vi "MDAQ_WRITE.vi"(8 "error in":errorcluster, 9 "ARG":string, 10 "CMD":string, 11 "VISA resource name":refnum<visa-resource-name>) -> (0 "error out":errorcluster, 3 "VISA resource name out":refnum<visa-resource-name>)   [LabVIEW 2021]
uses:
  e2ee38f0-3462-4155-9d7d-371542cbdf2c.vi
  e0b7c9b4-ca0d-4614-8169-0355f0fe5c3c.vi
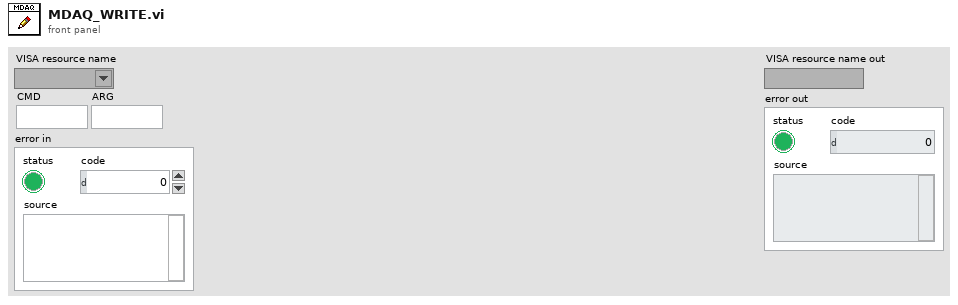
[diagram p1: front panel]
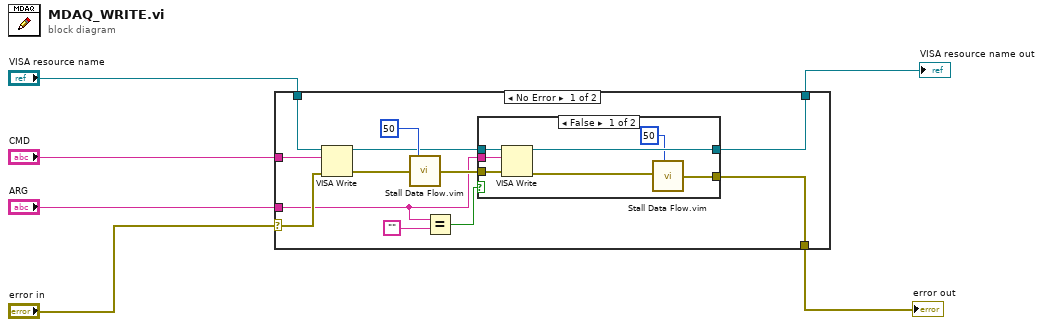
[diagram p0: block diagram]
diagram:
  n1 = case shown="No Error" "error in" {
    selector: "error in" -> [w12 w28]
    tunnel: "VISA resource name" -> [w18 w29]
    tunnel: "CMD" -> [w17 _]
    tunnel: "ARG" -> [w11 _]
    tunnel: [w8 w29] -> w3
    tunnel: [w7 w28] -> w2
    frame No Error {
      n2 = VISA Write(VISA resource name=w18, write buffer=w17, error in (no error)=w12) -> (VISA resource name out=w14:refnum<visa-resource-name>, error out=w16:errorcluster)  [unwired: 1 out]
      n3 = call "Stall Data Flow.vim"("value in"=w16, "milliseconds to wait"=u32 50) -> ("value out"=w13:errorcluster)  [unwired: 1 out]
      n4 = Equal?(x=w11, y="") -> (x = y?=w9:bool)
      n5 = case shown="False" w9 {
        tunnel: w14 -> [w25 w27]
        tunnel: w13 -> [w24 w26]
        tunnel: w11 -> [w23 _]
        tunnel: [w22 w27] -> w8
        tunnel: [w19 w26] -> w7
        frame False {
          n6 = VISA Write(VISA resource name=w25, write buffer=w23, error in (no error)=w24) -> (VISA resource name out=w22:refnum<visa-resource-name>, error out=w21:errorcluster)  [unwired: 1 out]
          n7 = call "Stall Data Flow.vim"("value in"=w21, "milliseconds to wait"=u32 50) -> ("value out"=w19:errorcluster)  [unwired: 1 out]
        }
        frame True {
        }
      }
    }
    frame Error {
    }
  }
  "VISA resource name out" <- w3
  "error out" <- w2
